vi "HHMI - Count with rollover U16.vi"(5 "Threshold\n(output will never be\nthis number or higher)":u16, 7 "Reset?":bool, 10 "Increment?":bool) -> (2 "total # counted\n(Reset occurs \nprior to Increment)":u16)   [LabVIEW 2012]
doc: "Counts up. Reset returns count to zero. Increment occurs after Reset."
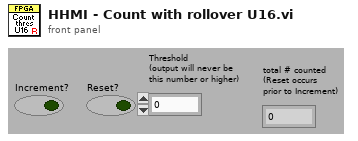
[diagram p1: front panel]
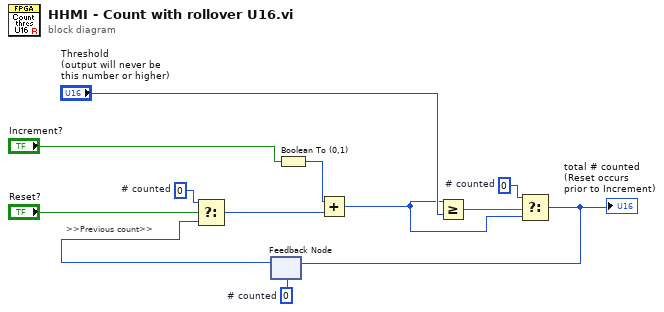
[diagram p0: block diagram]
diagram:
  w7 = u16 0  # # counted
  w9 = u16 0  # # counted
  w12 = u16 0  # # counted
  # ">>Previous count>>"
  n1 = feedback #1(w12) -> (w10:u16)
  n2 = Select(t=w9, s="Reset?", f=w10) -> (s? t:f=w3:u16)
  n3 = Boolean To (0,1)(Boolean="Increment?") -> (0, 1=w2:i16)
  n4 = Add(x=w2, y=w3) -> (x+y=w1:u16)
  n5 = Greater Or Equal?(x=w1, y="Threshold\n(output will never be\nthis number or higher)") -> (x >= y?=w6:bool)
  n6 = Select(t=w7, s=w6, f=w1) -> (s? t:f=w5:u16)
  "total # counted\n(Reset occurs \nprior to Increment)" <- w5
  n7 = feedback-in #1(w5) -> ()
